vi "measVoltGlobVarsWrite.vi"(0 "measVoltPulseLength(25ns)":i32, 2 "measVoltTimeout(10ns)":i32, 4 "timedOutWhileHandshake":bool, 5 "measVoltState":T2, 9 "writeMeasVoltCompleteDest":bool, 10 "writeOnlyMeasVoltState":bool, 11 "measVoltCompleteDest":T1, 18 "stopVoltMeas":bool caption="measVoltStop", 19 "writeStopVoltMeas":bool) -> ()   [LabVIEW 2014]
uses:
  Controls/measVoltState.ctl
  Controls/measVoltCompleteDest.ctl
  <vilib>/rvi/Emulation/niFpgaSctlEmulationGetInTimedLoop.vi
  measVoltGlobVars.vi
  <vilib>/rvi/Emulation/niFpgaProcessEmulError.vi
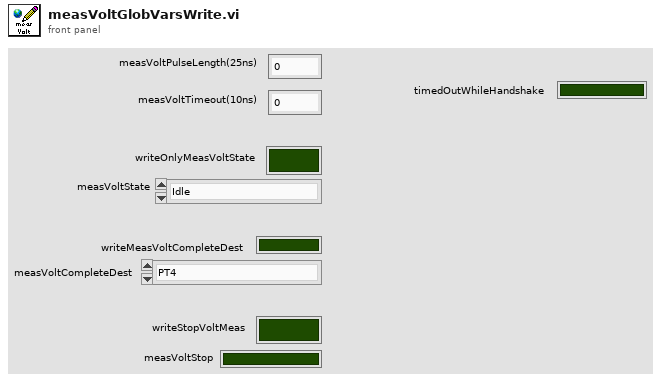
[diagram p1: front panel]
types:
  T1 = typedef "measVoltCompleteDest.ctl" = enum16{"PT4", "C1D30", "C1D31", "PT4_C1D30", "PT4_C1D31", "PT4_C1D30_C1D31", "C1D30_C1D31", "software"}
  T2 = typedef "measVoltState.ctl" = enum16{"Idle", "sendMeasRequest", "waitUntilDone", "done"}
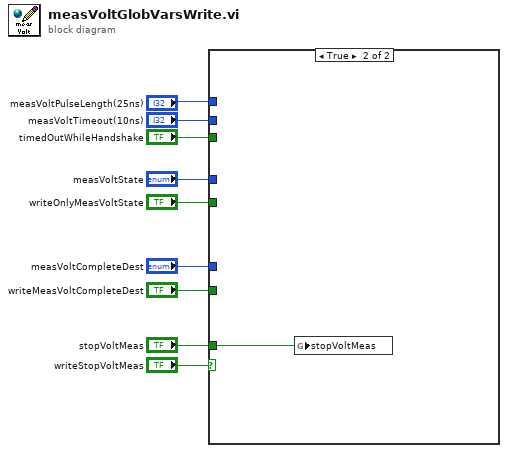
[diagram p0: block diagram]
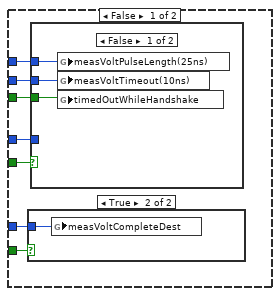
[diagram p2: hidden frame]
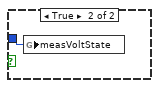
[diagram p4: hidden frame]
diagram:
  n1 = case shown="True" "writeStopVoltMeas" {
    tunnel: "measVoltState" -> [w16 _]
    tunnel: "writeOnlyMeasVoltState" -> [w15 _]
    tunnel: "timedOutWhileHandshake" -> [w14 _]
    tunnel: "measVoltTimeout(10ns)" -> [w13 _]
    tunnel: "measVoltPulseLength(25ns)" -> [w12 _]
    tunnel: "measVoltCompleteDest" -> [w11 _]
    tunnel: "writeMeasVoltCompleteDest" -> [w10 _]
    tunnel: "stopVoltMeas" -> [_ w22]
    frame False {
      n2 = case shown="True" w10 {
        tunnel: w11 -> [_ w17]
        frame False {
        }
        frame True {
          n3 = global write "measVoltGlobVars.vi" "measVoltCompleteDest"(w17) -> ()
        }
      }
      n4 = case shown="False" w15 {
        tunnel: w16 -> [_ w21]
        tunnel: w14 -> [w20 _]
        tunnel: w13 -> [w19 _]
        tunnel: w12 -> [w18 _]
        frame False {
          n5 = global write "measVoltGlobVars.vi" "measVoltPulseLength(25ns)"(w18) -> ()
          n6 = global write "measVoltGlobVars.vi" "measVoltTimeout(10ns)"(w19) -> ()
          n7 = global write "measVoltGlobVars.vi" "timedOutWhileHandshake"(w20) -> ()
        }
        frame True {
          n8 = global write "measVoltGlobVars.vi" "measVoltState"(w21) -> ()
        }
      }
    }
    frame True {
      n9 = global write "measVoltGlobVars.vi" "stopVoltMeas"(w22) -> ()
    }
  }
